vi "deleteTupla.vi"(8 "error in":errorcluster, 10 "table":string, 11 "RawIndexToModify":i32[](array[numeric])) -> (0 "error out":errorcluster)   [LabVIEW 2014]
uses:
  <vilib>/addons/database/Connection.llb/DB Tools Open Connec (String).vi
  <vilib>/addons/database/NI_Database_API.lvlib
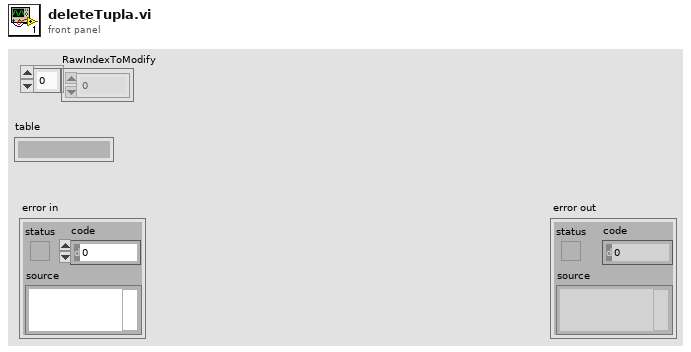
[diagram p1: front panel]
types:
  T1 = typedef "NI_Database_API.lvlib/Conn ObjectReference.ctl" = refnum<k1>
  T2 = typedef "NI_Database_API.lvlib/DB Tools DataTypes.ctl" = enum16{"String", "Long (I32)", "Single (SGL)", "Double (DBL)", "Date/Time", "Binary"}
  T3 = cluster{"name":string, "database data type":T2, "defined size":i32}[]
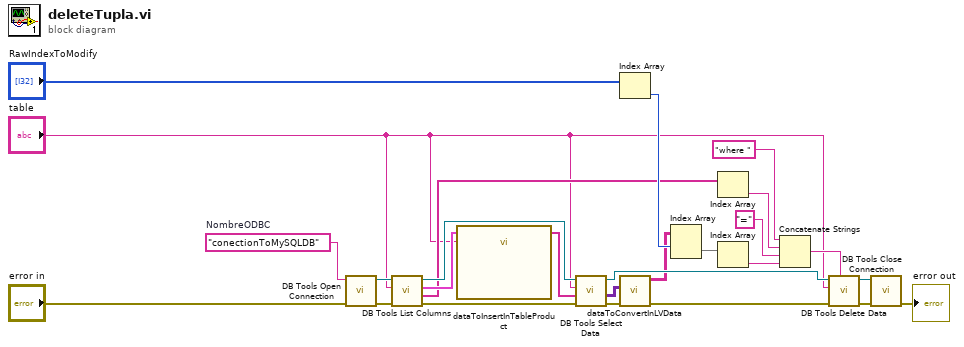
[diagram p0: block diagram]
diagram:
  w18 = "conectionToMySQLDB"  # NombreODBC
  n1 = call-poly <vilib>:"DB Tools Open Connection.vi"("error in (no error)"="error in", "connection information"=w18) -> ("error out"=w10:errorcluster, "connection reference"=w11:T1)  [unwired: 6 in]
  n2 = call <vilib>:"DB Tools List Columns.vi"("error in (no error)"=w10, "table"="table", "connection reference"=w11) -> ("error out"=w14:errorcluster, "columns"=w5:string[], "column information"=w12:T3, "connection reference out"=w13:T1)  [unwired: 1 in]
  n3 = call "dataToInsertInTableProduct.vi"("arrayNamesInTableIN"=w12, "tableIn"="table") -> ("arrayNamesInTableOUT"=w16:string[])  [unwired: 7 in, 6 out]
  n4 = call <vilib>:"DB Tools Select Data.vi"("error in (no error)"=w14, "columns"=w16, "table"="table", "connection reference"=w13) -> ("error out"=w9:errorcluster, "data"=w15:variant[][], "connection reference out"=w8:T1)  [unwired: 2 in]
  n5 = Index Array(array="RawIndexToModify") -> (element=w20:i32)  [unwired: 1 in]
  n6 = call "dataToConvertInLVData.vi"("error in"=w9, "dataReadingIn"=w15) -> ("error out"=w7:errorcluster, "dataReadingOut"=w6:string[][])  [unwired: 8 in]
  n7 = Index Array(array=w6, index (row)=w20) -> (element=w21:string[])  [unwired: 1 in]
  n8 = Index Array(array=w5) -> (element=w24:string)  [unwired: 1 in]
  n9 = Index Array(array=w21) -> (element=w25:string)  [unwired: 1 in]
  n10 = Concatenate Strings("where " ("condition"), w24, "=" ("string"), w25) -> (w26:string)
  n11 = call <vilib>:"DB Tools Delete Data.vi"("condition"=w26, "error in (no error)"=w7, "table"="table", "connection reference"=w8) -> ("error out"=w3:errorcluster, "connection reference out"=w2:T1)  [unwired: 6 in]
  n12 = call <vilib>:"DB Tools Close Connection.vi"("error in (no error)"=w3, "connection reference"=w2) -> ("error out"=→"error out":errorcluster)  [unwired: 5 in]
